vi "_Chip Select.vi"(7 "ChipType":T1) -> ()   [LabVIEW 2015]
uses:
  Type/_FPGA Chip Type.ctl
  <vilib>/rvi/eio/common/nirviEmuTemplateMethod_errors.vi
  <vilib>/eio/EIONode/EIONode.xnode
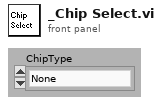
[diagram p1: front panel]
types:
  T1 = typedef "_FPGA Chip Type.ctl" = enum8{"None", "ADC1", "ADC2", "ADC3", "ADC4", "ADC5", "ADC6", "ADC7", "ADC8", "ADC9", "ADC10", "ADC11", "ADC12", "ADC13", "DAC1", "DAC2", "DAC3", "DAC4", "DAC5", "LENS1", "LENS2", "LENS3", "LENS4", "LENS5", "LENS6", "LENS7", "MASS1", "MASS2", "MASS3", "MASS4", "MASS5", "OSC1", "OSC2", "OSC3", "LATCH1", "LATCH2", "LATCH3", "LATCH4", "PIC1", "PIC2", "PIC3", "PIC4"}
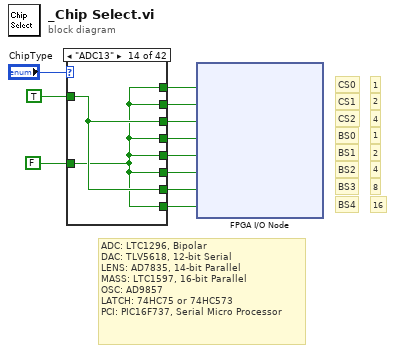
[diagram p0: block diagram]
diagram:
  # "8"
  # "16"
  # "4"
  # "2"
  # "1"
  # "4"
  # "2"
  # "1"
  # "BS3"
  # "BS4"
  # "BS2"
  # "BS1"
  # "ADC: LTC1296, Bipolar\nDAC: TLV5618, 12-bit Serial\nLENS: AD7835, 14-bit Parallel\nMASS: LTC1597, 16-bit Parallel\nOSC: AD9857\nLATCH: 74HC75 or 74HC573\nPCI: PIC16F737, Serial Micro Processor"
  # "BS0"
  # "CS2"
  # "CS1"
  # "CS0"
  n1 = case shown="\"ADC13\"" "ChipType" {
    tunnel: TRUE -> [w13 w14 w17 w19 w21 w22 w24 w27 w29 w30 w33 w34 w36 w39 w41 w43 w45 w47 w48 w51 w53 w54 w57 w58 w61 w62 w65 w66 w68 w70 w73 w74 w76 w78 w81 w83 w85 w87 w89 w90 w93 w94]
    tunnel: FALSE -> [w12 w15 w16 w18 w20 w23 w25 w26 w28 w31 w32 w35 w37 w38 w40 w42 w44 w46 w49 w50 w52 w55 w56 w59 w60 w63 w64 w67 w69 w71 w72 w75 w77 w79 w80 w82 w84 w86 w88 w91 w92 w95]
    tunnel: [w13 w14 w16 w18 w20 w22 w24 w26 w28 w30 w32 w34 w37 w38 w41 w42 w44 w46 w48 w50 w52 w54 w56 w58 w60 w62 w65 w66 w68 w70 w72 w74 w76 w78 w80 w82 w84 w86 w88 w90 w92 w94] -> w10
    tunnel: [w13 w15 w16 w19 w21 w23 w25 w27 w29 w31 w33 w35 w36 w39 w40 w42 w44 w46 w49 w50 w52 w55 w56 w59 w60 w63 w64 w67 w69 w71 w72 w74 w76 w78 w81 w83 w85 w87 w88 w91 w92 w95] -> w9
    tunnel: [w13 w14 w16 w18 w20 w22 w24 w26 w28 w30 w32 w35 w37 w38 w40 w43 w45 w47 w48 w50 w52 w55 w56 w59 w60 w63 w64 w67 w69 w71 w73 w75 w77 w79 w81 w82 w84 w86 w88 w91 w92 w95] -> w8
    tunnel: [w12 w14 w16 w18 w21 w23 w25 w27 w29 w31 w32 w35 w37 w38 w41 w43 w44 w46 w49 w50 w52 w55 w56 w59 w60 w63 w65 w66 w68 w71 w72 w74 w76 w78 w80 w83 w84 w87 w89 w90 w92 w95] -> w5
    tunnel: [w12 w15 w17 w18 w20 w22 w25 w26 w28 w30 w33 w34 w36 w38 w40 w42 w45 w46 w49 w50 w53 w54 w56 w59 w61 w62 w64 w67 w69 w71 w72 w75 w77 w79 w80 w83 w84 w86 w89 w90 w92 w95] -> w4
    tunnel: [w12 w15 w16 w19 w21 w22 w25 w26 w29 w30 w33 w35 w36 w38 w40 w42 w45 w46 w48 w51 w53 w54 w56 w59 w61 w62 w64 w66 w68 w70 w73 w75 w76 w78 w81 w82 w85 w86 w88 w91 w93 w94] -> w3
    tunnel: [w12 w15 w16 w18 w20 w23 w24 w27 w29 w30 w33 w35 w37 w39 w40 w42 w44 w47 w49 w50 w52 w55 w57 w58 w61 w62 w65 w67 w68 w71 w72 w74 w77 w78 w80 w83 w85 w86 w89 w90 w93 w94] -> w2
    tunnel: [w12 w15 w16 w18 w20 w23 w25 w26 w28 w31 w32 w35 w37 w38 w40 w42 w44 w46 w49 w50 w52 w55 w56 w59 w60 w63 w64 w67 w69 w71 w72 w75 w77 w79 w80 w82 w84 w86 w88 w91 w92 w95] -> w1
    frame "None", Default {
    }
    frame "ADC1" {
    }
    frame "ADC2" {
    }
    frame "ADC3" {
    }
    frame "ADC4" {
    }
    frame "ADC5" {
    }
    frame "ADC6" {
    }
    frame "ADC7" {
    }
    frame "ADC8" {
    }
    frame "ADC9" {
    }
    frame "ADC10" {
    }
    frame "ADC11" {
    }
    frame "ADC12" {
    }
    frame "ADC13" {
    }
    frame "DAC1" {
    }
    frame "DAC2" {
    }
    frame "DAC3" {
    }
    frame "DAC4" {
    }
    frame "DAC5" {
    }
    frame "LENS1" {
    }
    frame "LENS2" {
    }
    frame "LENS3" {
    }
    frame "LENS4" {
    }
    frame "LENS5" {
    }
    frame "LENS6" {
    }
    frame "LENS7" {
    }
    frame "MASS1" {
    }
    frame "MASS2" {
    }
    frame "MASS3" {
    }
    frame "MASS4" {
    }
    frame "MASS5" {
    }
    frame "OSC1" {
    }
    frame "OSC2" {
    }
    frame "OSC3" {
    }
    frame "LATCH1" {
    }
    frame "LATCH2" {
    }
    frame "LATCH3" {
    }
    frame "LATCH4" {
    }
    frame "PIC1" {
    }
    frame "PIC2" {
    }
    frame "PIC3" {
    }
    frame "PIC4" {
    }
  }
  n2 = xnode "FPGA I/O Node"("Digtal IO/DIO22"=w10, "Digtal IO/DIO21"=w8, "Digtal IO/DIO20"=w9, "Digtal IO/DIO19"=w5, "Digtal IO/DIO17"=w4, "Digtal IO/DIO16"=w3, "Digtal IO/DIO15"=w2, "Digtal IO/DIO14"=w1) -> ()  [unwired: 8 in, 8 out]
